vi "OphirAcquire_v2.vi"(0 "Instruments in":refnum<class "Instruments.lvclass">, 1 "Type":T1, 2 "error in (no error)":errorcluster) -> (3 "Instruments out":refnum<class "Instruments.lvclass">, 4 "Power,uW":dbl, 5 "Remeasure?":bool, 6 "error out":errorcluster)   [LabVIEW 2012, in "Instruments.lvclass"]
uses:
  Instruments.lvclass
  Controls/SpectrometerOphirSelector.ctl
  Instruments.lvclass/Instruments.ctl
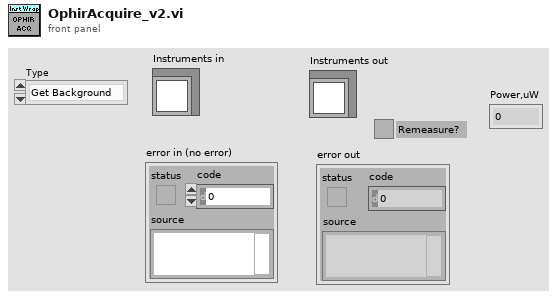
[diagram p1: front panel]
types:
  T1 = typedef "SpectrometerOphirSelector.ctl" = enum16{"Get Background", "Measure", "Measure50", "Raw"}
  T2 = typedef "OphirRef.ctl" = cluster{"OphirComRef":refnum<k7>, "deviceHandle":i32, "Channel":i32, "SerialNumber":string, "Background Wl":dbl, "Background":dbl, "CalWl":dbl}
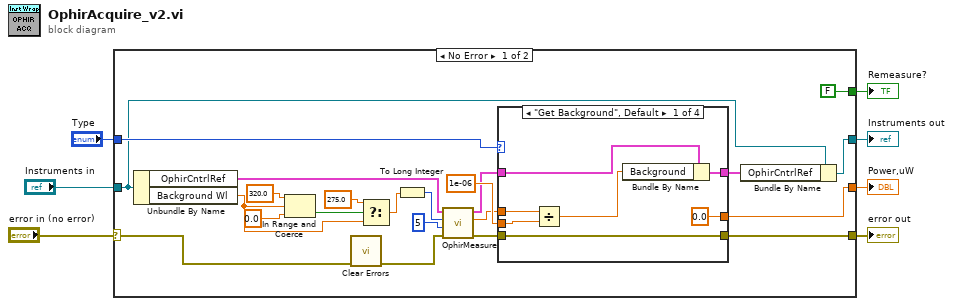
[diagram p0: block diagram]
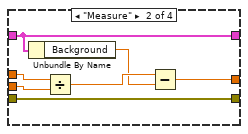
[diagram p2: hidden frame]
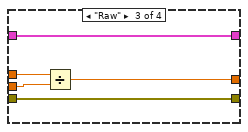
[diagram p3: hidden frame]
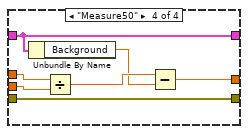
[diagram p4: hidden frame]
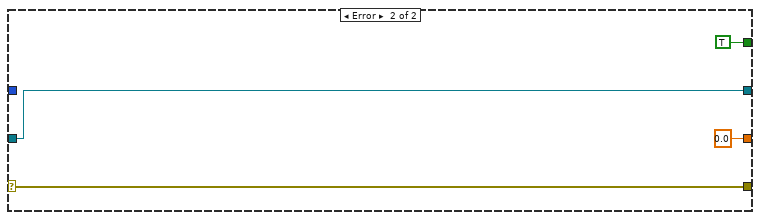
[diagram p5: hidden frame]
diagram:
  n1 = case shown="No Error" "error in (no error)" {
    selector: "error in (no error)" -> [w9 w59]
    tunnel: [w17 w59] -> w6
    tunnel: "Instruments in" -> [w21 w57]
    tunnel: "Type" -> [w29 _]
    tunnel: [w28 0.0] -> w2
    tunnel: [FALSE TRUE] -> w3
    tunnel: [w19 w57] -> w1
    frame No Error {
      n2 = Unbundle By Name(w21) -> ("OphirCntrlRef"=w26:T2, "Background Wl"=w12:dbl)
      n3 = In Range and Coerce(upper limit=320.0, x=w12, lower limit=0.0) -> (In Range?=w13:bool)  [unwired: 1 out]
      n4 = call <vilib>:"Clear Errors.vi"("error in (no error)"=w9) -> ("error out"=w8:errorcluster)  [unwired: 6 in]
      n5 = Select(t=275.0, s=w13, f=w12) -> (s? t:f=w10:dbl)
      n6 = To Long Integer(number=w10) -> (32bit integer=w25:i32)
      n7 = call "OphirMeasure.vi"("error in (no error)"=w8, "Samples"=5, "wavelength"=w25, "OphirRef In"=w26) -> ("error out"=w18:errorcluster, "median"=w23:dbl, "OphirRef Out"=w22:T2)  [unwired: 1 out]
      n8 = case shown="\"Get Background\", Default" w29 {
        tunnel: [0.0 w41 w46 w51] -> w28
        tunnel: [w35 w39 w45 w50] -> w20
        tunnel: 1e-06 ("y") -> [w34 w40 w48 w53]
        tunnel: w23 -> [w31 w37 w47 w52]
        tunnel: w22 -> [w32 w39 w45 w50]
        tunnel: w18 -> [w30 w38 w44 w49]
        tunnel: [w30 w38 w44 w49] -> w17
        frame "Get Background", Default {
          n9 = Divide(x=w31, y=w34) -> (x/y=w36:dbl)
          n10 = Bundle By Name(cluster=w32, "Background"=w36) -> (w35:T2)
        }
        frame "Measure" {
          n11 = Unbundle By Name(w39) -> ("Background"=w42:dbl)
          n12 = Divide(x=w37, y=w40) -> (x/y=w43:dbl)
          n13 = Subtract(x=w43, y=w42) -> (x-y=w41:dbl)
        }
        frame "Raw" {
          n14 = Divide(x=w47, y=w48) -> (x/y=w46:dbl)
        }
        frame "Measure50" {
          n15 = Unbundle By Name(w50) -> ("Background"=w54:dbl)
          n16 = Divide(x=w52, y=w53) -> (x/y=w55:dbl)
          n17 = Subtract(x=w55, y=w54) -> (x-y=w51:dbl)
        }
      }
      n18 = Bundle By Name(cluster=w21, "OphirCntrlRef"=w20) -> (w19:refnum<class "Instruments.lvclass">)
    }
    frame Error {
    }
  }
  "error out" <- w6
  "Instruments out" <- w1
  "Power,uW" <- w2
  "Remeasure?" <- w3
